vi "ClearOverload.vi"() -> (0 "Error Out":errorcluster, 1 "min wait time (ms)":u32=250000000)   [LabVIEW 2015]
doc: "Configures device parameters for an NI 5170/5171"
uses:
  OscopeAPI/Device Session.lvclass
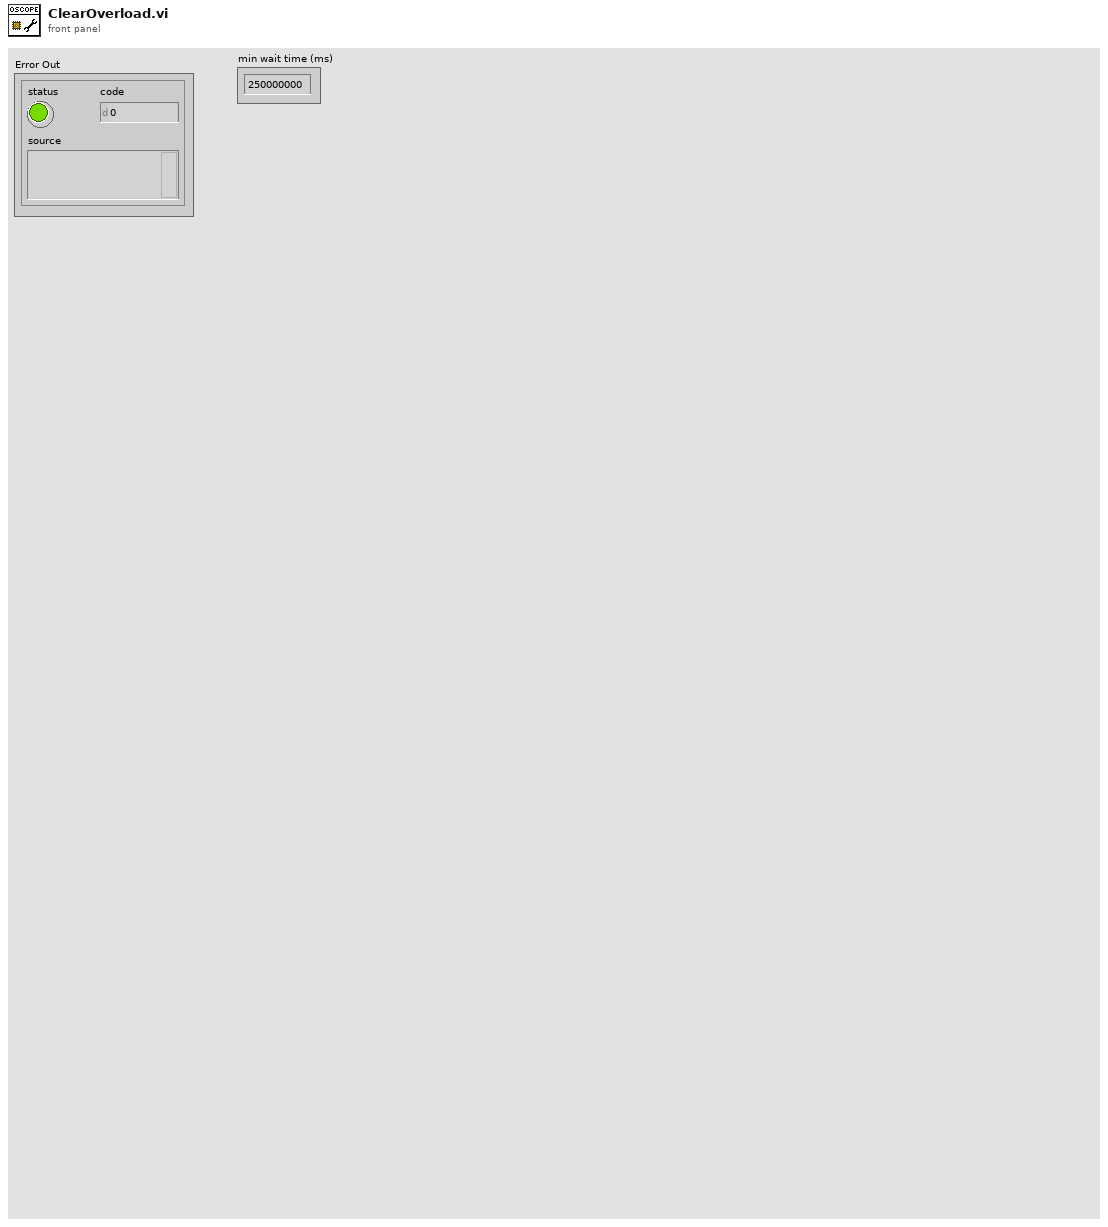
[diagram p1: front panel]
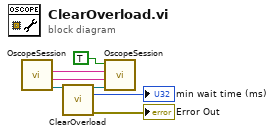
[diagram p0: block diagram]
diagram:
  n1 = call "OscopeSession.vi"() -> ("Session Out"=w4:refnum<class "Device Session.lvclass">, "Bitfile Path Out"=w2:string, "Device Address Out"=w3:string)  [unwired: 9 in]
  n2 = call "ClearOverload.vi"("device session in"=w4) -> ("device session out"=w6:refnum<class "Device Session.lvclass">, "min wait time (ms)"=→"min wait time (ms)":u32, "error out"=→"Error Out":errorcluster)  [unwired: 12 in]
  n3 = call "OscopeSession.vi"("Session In"=w6, "Bitfile Path In"=w2, "Device Address In"=w3, "Write"=TRUE) -> ()  [unwired: 5 in, 3 out]
